vi "Set Panel Visibility.vi"(8 "error in (no error)":errorcluster, 10 "Visible":bool, 11 "Panel In":refnum<class "Panel.lvclass">) -> (0 "error out":errorcluster, 3 "Panel":refnum<class "Panel.lvclass">)   [LabVIEW 2018]
uses:
  Panel/Panel.lvclass
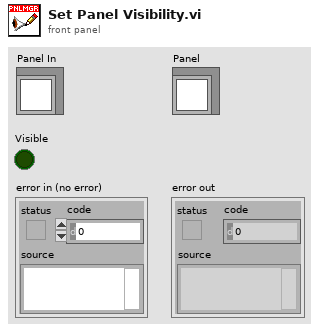
[diagram p1: front panel]
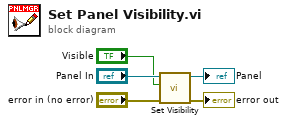
[diagram p0: block diagram]
diagram:
  n1 = call "Set Visibility.vi"("error in (no error)"="error in (no error)", "Visible"="Visible", "Panel in"="Panel In") -> ("error out"=→"error out":errorcluster, "Panel out"=→"Panel":refnum<class "Panel.lvclass">)  [unwired: 7 in]
